vi "Update Latest Broadcast Data.vi"(8 "error in (no error)":errorcluster, 10 "Latest Messages":map{string, refnum<class "Debug Data.lvclass">}(c390), 11 "List Seen Processes View Model In":refnum<class "Process Tree View Model.lvclass">) -> (0 "error out":errorcluster, 3 "List Seen Processes View Model Out":refnum<class "Process Tree View Model.lvclass">)   [LabVIEW 2020, in "Process Tree View Model.lvclass"]
uses:
  Process Tree View Model.lvclass
  Process Tree View Model.lvclass/Process Tree View Model.ctl
  Debug Data/Debug Data.lvclass
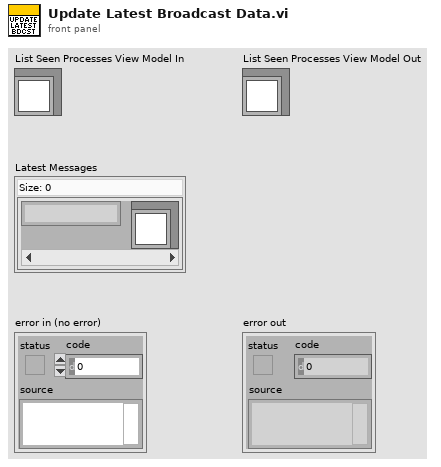
[diagram p1: front panel]
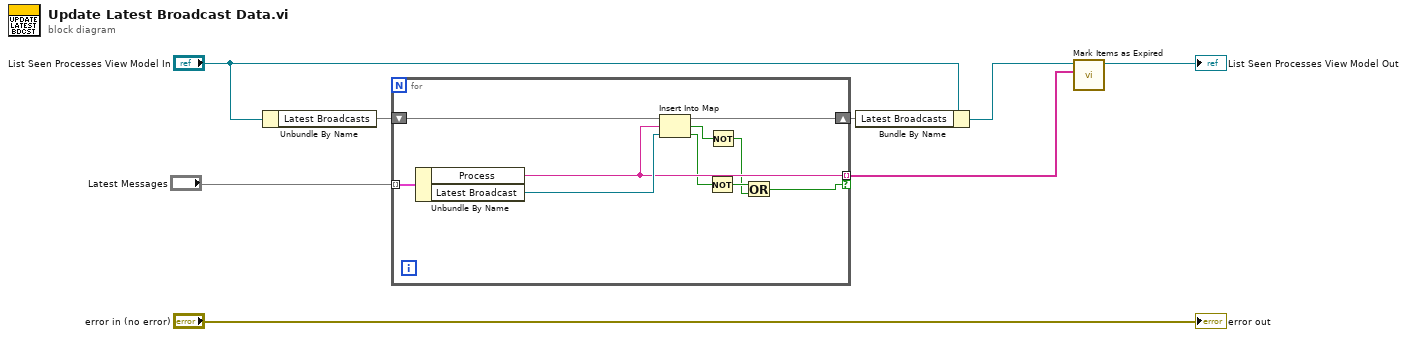
[diagram p0: block diagram]
diagram:
  n1 = Unbundle By Name("List Seen Processes View Model In") -> ("Latest Broadcasts"=w6:map{string, refnum<class "Debug Data.lvclass">})
  n2 = for {
    shift-right: [w15] -> w5
    shift-left: w6 -> [w17]
    tunnel: "Latest Messages" -> [w18] mode=indexing
    tunnel: [w14] -> w2 mode=indexing if=w13
    n3 = Unbundle By Name(w18) -> ("Process"=w14:string, "Latest Broadcast"=w16:refnum<class "Debug Data.lvclass">)
    n4 = Insert Into Map(map in=w17, key=w14, value=w16) -> (map out=w15:map{string, refnum<class "Debug Data.lvclass">}, key already included?=w10:bool, value unchanged?=w12:bool)
    n5 = Not(x=w12) -> (.not. x?=w11:bool)
    n6 = Not(x=w10) -> (.not. x?=w9:bool)
    n7 = Or(x=w11, y=w9) -> (x .or. y?=w13:bool)
  }
  n8 = Bundle By Name(cluster="List Seen Processes View Model In", "Latest Broadcasts"=w5) -> (w4:refnum<class "Process Tree View Model.lvclass">)
  n9 = call "Mark Items as Expired.vi"("Expired Tags"=w2, "Process Tree View Model in"=w4) -> ("Process Tree View Model out"=→"List Seen Processes View Model Out":refnum<class "Process Tree View Model.lvclass">)  [unwired: 9 in]
  "error out" <- "error in (no error)"
